vi "user defined.vi"(6 "timeout (25000ms)":i32=25000, 8 "error in (no error)":errorcluster, 9 "parameters":string[](array[string]), 10 "command":string, 11 "daemon reference in":refnum<k5>) -> (0 "error out":errorcluster, 2 "response":string, 3 "daemon reference out":refnum<k5>, 4 "parameter(s) out":string, 5 "command out":string)   [LabVIEW 2017]
doc: "<b>Command: </b>Anything\n\n<b>Description: </b> This command can be used to send a \"user defined\" command and set of parameters.\n\n<b>Parameters: </b> Anything\n____________________________________________\nDIPC 692 Daemon API 10.0.0.1\nSam Tee - Dyson Technology Ltd\nCopyright (c) 2024, Dyson Technology Ltd"
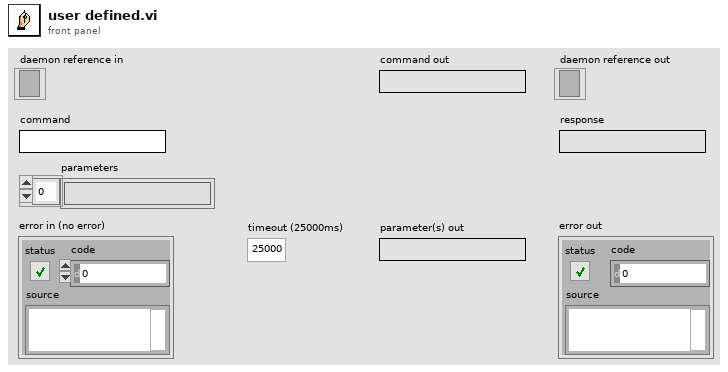
[diagram p1: front panel]
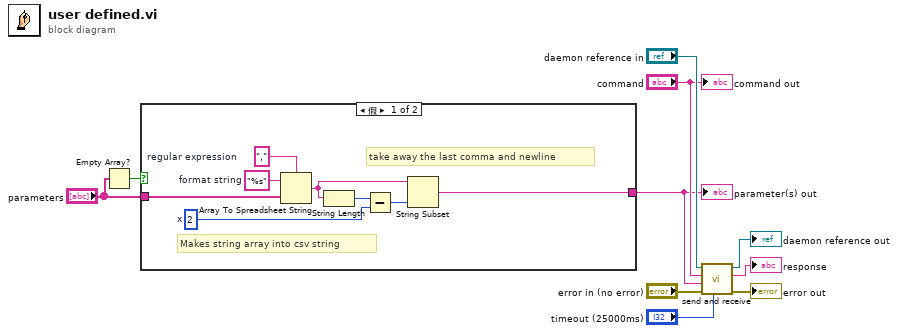
[diagram p0: block diagram]
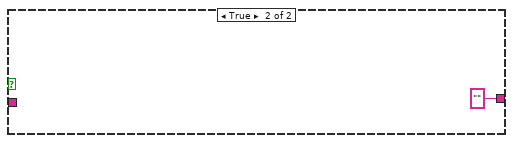
[diagram p2: hidden frame]
diagram:
  n1 = Empty Array?(array="parameters") -> (empty?=w3:bool)
  n2 = case shown="假" w3 {
    tunnel: [w12 ""] -> w2
    tunnel: "parameters" -> [w11 _]
    frame False {
      w18 = ","  # regular expression
      w17 = 2  # x
      w13 = "%s"  # format string
      # "Makes string array into csv string"
      # "take away the last comma and newline"
      n3 = Array To Spreadsheet String(delimiter (Tab)=w18, array=w11, 3:w13) -> (spreadsheet string=w16:string)
      n4 = String Length(string=w16) -> (length=w14:i32)
      n5 = Subtract(x=w14, y=w17) -> (x-y=w15:i32)
      n6 = String Subset(string=w16, length (rest)=w15) -> (substring=w12:string)  [unwired: 1 in]
    }
    frame True {
    }
  }
  "parameter(s) out" <- w2
  n7 = call "send and receive.vi"("timeout (25000ms)"="timeout (25000ms)", "error in (no error)"="error in (no error)", "data"=w2, "command"="command", "daemon reference in"="daemon reference in") -> ("error out"=→"error out":errorcluster, "response"=→"response":string, "daemon reference out"=→"daemon reference out":refnum<k5>)  [unwired: 4 in]
  "command out" <- "command"
